vi "Teleop.vi"(10 "Match Info":T1={"Autonomous Elapsed Seconds"=0.0, "TeleOp Elapsed Seconds"=0.0, "Disabled Elapsed Seconds"=0.0, "Visited Autonomous"=FALSE, "Visited TeleOp"=FALSE, "Visited Disabled"=FALSE, "Autonomous Settings"={"Autonomous Style"=enum."Independent", "VI Refnum"=refnum}}, 11 "Call Context":T2) -> ()   [LabVIEW 2014]
doc: "This VI is called for each TeleOp packet received from the DS where the robot is not disabled. It is often used to read from the joysticks and update I/O or to update setpoints for timed control loops. It should complete and return within 20 milliseconds or it may miss DS packets."
uses:
  <vilib>/Rock Robotics/WPI/DriverStation/WPI_DriverStationDerivedRobotMode.ctl
  <vilib>/Rock Robotics/WPI/DriverStation/WPI_DriverStationMatch Info.ctl
  <vilib>/Rock Robotics/WPI/RobotDrive/WPI_RobotDriveGetSetRefNum.vi
  <vilib>/Rock Robotics/WPI/Joystick/WPI_JoystickGetSetRefNum.vi
  <vilib>/Rock Robotics/Network Tables/SD Write Boolean Array.vi
  <vilib>/Rock Robotics/Network Tables/SD Write Numeric Array.vi
  <vilib>/Rock Robotics/Network Tables/SD Write Number.vi
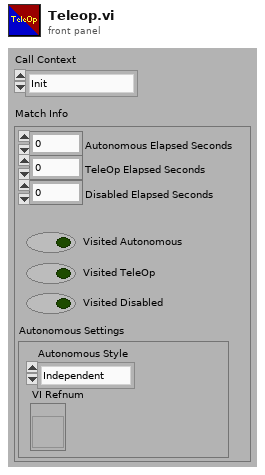
[diagram p1: front panel]
types:
  T1 = typedef "WPI_DriverStationMatch Info.ctl" = cluster{"Autonomous Elapsed Seconds":dbl, "TeleOp Elapsed Seconds":dbl, "Disabled Elapsed Seconds":dbl, "Visited Autonomous":bool, "Visited TeleOp":bool, "Visited Disabled":bool, "Autonomous Settings":cluster{"Autonomous Style":enum16{"Iterative", "Independent"}, "VI Refnum":refnum<vi>}}
  T2 = typedef "WPI_DriverStationDerivedRobotMode.ctl" = enum16{"Init", "Execute", "Stop"}
  T3 = typedef "WPI_MotorControlDeviceRef.ctl" = cluster{"DeviceStatus":errorcluster, "Type":T4, "PWM":cluster{"Controller":T5, "PWM Channel":T6, "DeadBand":T7}, "CAN":cluster{"Device Number":u8, "Control Mode":T8, "Semaphore":T9, "Max Vout":dbl, "TalonSRX Control Mode":T10}, "Invert":bool, "TransformRef":T11, "InvTransformRef":T11}
  T4 = typedef "WPI_MotorControlType.ctl" = enum16{"PWM", "CAN", "CANTalonSRX"}
  T5 = typedef "FPGA_TypedefDigitalModule.ctl" = enum16{"Controller 1"}
  T6 = typedef "FPGA_DIOPWMChannel.ctl" = enum8{"PWM 0", "PWM 1", "PWM 2", "PWM 3", "PWM 4", "PWM 5", "PWM 6", "PWM 7", "PWM 8", "PWM 9", "PWM MXP 0", "PWM MXP 1", "PWM MXP 2", "PWM MXP 3", "PWM MXP 4", "PWM MXP 5", "PWM MXP 6", "PWM MXP 7", "PWM MXP 8", "PWM MXP 9", "Invalid"}
  T7 = typedef "WPI_PWMDeadband.ctl" = cluster{"Name":string, "maxPositivePwm":i32, "minPositivePwm":i32, "centerPwm":i32, "maxNegativePwm":i32, "minNegativePwm":i32, "angularRange":u16}
  T8 = typedef "WPI_CANJaguar_ControlMode.ctl" = enum8{"Percent VBus", "Current", "Speed", "Position", "Voltage"}
  T9 = typedef "Semaphore RefNum" = refnum<k1>
  T10 = typedef "WPI_CANTalonSRX_APIControlMode.ctl" = enum8{"Percent VBus", "Speed", "Position", "Slave", "Unchanged / Invalid"}
  T11 = typedef "WPI_PWMTransform_ConPane.ctl" = refnum<vi>
  T12 = typedef "WPI_JoystickDevRef.ctl" = cluster{"Device":T13}
  T13 = typedef "WPI_JoystickDeviceEnum.ctl" = enum16{"USB 0", "USB 1", "USB 2", "USB 3", "USB 4", "USB 5"}
  T14 = typedef "WPI_RobotDriveDevRef.ctl" = cluster{"DevStatus":errorcluster, "Motors[]":T3[], "Square Inputs":bool, "Max Output":dbl}
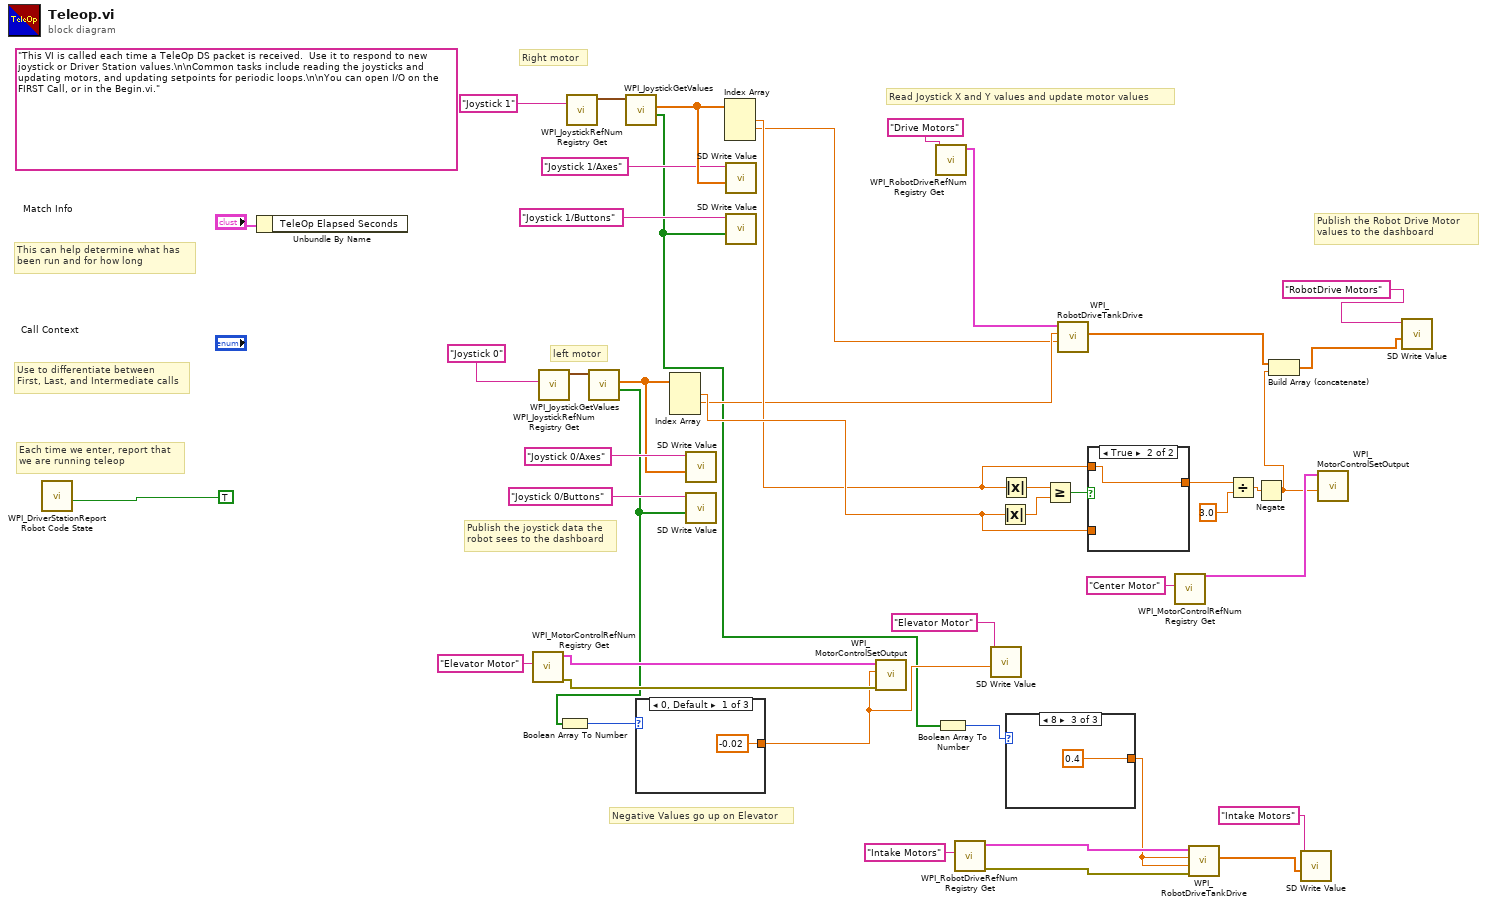
[diagram p0: block diagram]
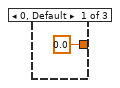
[diagram p2: hidden frame]
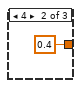
[diagram p3: hidden frame]
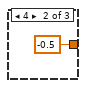
[diagram p4: hidden frame]
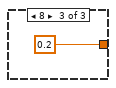
[diagram p5: hidden frame]
diagram:
  (unwired) "This VI is called each time a TeleOp DS packet is received.  Use it to respond to new joystick or Driver Station values.\n\nCommon tasks include reading the joysticks and updating motors, and updating setpoints for periodic loops.\n\nYou can open I/O on the FIRST Call, or in the Begin.vi."
  # "Negative Values go up on Elevator"
  # "left motor"
  # "Right motor"
  # "Publish the Robot Drive Motor\nvalues to the dashboard"
  # "Publish the joystick data the\nrobot sees to the dashboard"
  # "Each time we enter, report that\nwe are running teleop"
  # "Use to differentiate between\nFirst, Last, and Intermediate calls"
  # "This can help determine what has\nbeen run and for how long"
  # "Read Joystick X and Y values and update motor values"
  n1 = call <vilib>:"WPI_DriverStationReport Robot Code State.vi"("TeleOp"=TRUE ("Autonomous")) -> ()  [unwired: 10 in, 1 out]
  n2 = Unbundle By Name("Match Info") -> ()  [unwired: 1 out]
  n3 = call <vilib>:"WPI_MotorControlRefNum Registry Get.vi"("refnum name"="Elevator Motor") -> ("error out"=w19:errorcluster, "MotorControlDevRef"=w20:T3)  [unwired: 9 in]
  n4 = call <vilib>:"WPI_JoystickRefNum Registry Get.vi"("refnum name"="Joystick 0") -> ("JoystickDevRef"=w36:T12)  [unwired: 1 in, 9 out]
  n5 = call <vilib>:"WPI_JoystickRefNum Registry Get.vi"("refnum name"="Joystick 1") -> ("JoystickDevRef"=w31:T12)  [unwired: 9 in, 1 out]
  n6 = call <vilib>:"WPI_JoystickGetValues.vi"("JoystickDevRef"=w36) -> ("Buttons"=w18:bool[], "Axes"=w38:dbl[])  [unwired: 6 in, 3 out]
  n7 = Boolean Array To Number(Boolean array=w18) -> (number=w17:u32)
  n8 = call <vilib>:"WPI_JoystickGetValues.vi"("JoystickDevRef"=w31) -> ("Buttons"=w5:bool[], "Axes"=w35:dbl[])  [unwired: 6 in, 3 out]
  n9 = case shown="0, Default" w17 {
    tunnel: [-0.02 ("Output") -0.5 ("Output") 0.2 ("Output")] -> w15
    frame 0, Default {
    }
    frame 4 {
    }
    frame 8 {
    }
  }
  n10 = Index Array(array=w38) -> (element #1=w24:dbl, element #2=w14:dbl)  [unwired: 3 in, 1 out]
  n11 = call-poly <vilib>:"SD Write Value.vi"("Numeric Array"=w38, "Name"="Joystick 0/Axes") -> ()  [unwired: 8 in, 2 out]
  n12 = call-poly <vilib>:"SD Write Value.vi"("Boolean Array"=w18, "Name"="Joystick 0/Buttons") -> ()  [unwired: 8 in, 2 out]
  n13 = Index Array(array=w35) -> (element #1=w23:dbl, element #2=w13:dbl)  [unwired: 3 in, 1 out]
  n14 = call-poly <vilib>:"SD Write Value.vi"("Numeric Array"=w35, "Name"="Joystick 1/Axes") -> ()  [unwired: 8 in, 2 out]
  n15 = call-poly <vilib>:"SD Write Value.vi"("Boolean Array"=w5, "Name"="Joystick 1/Buttons") -> ()  [unwired: 8 in, 2 out]
  n16 = call <vilib>:"WPI_MotorControlSetOutput.vi"("error in (no error)"=w19, "Output"=w15, "MotorControlDevRef"=w20) -> ()  [unwired: 6 in, 3 out]
  n17 = call <vilib>:"WPI_RobotDriveRefNum Registry Get.vi"("refnum name"="Drive Motors") -> ("RobotDriveDevRef"=w22:T14)  [unwired: 1 in, 9 out]
  n18 = Boolean Array To Number(Boolean array=w5) -> (number=w4:u32)
  n19 = call <vilib>:"WPI_RobotDriveRefNum Registry Get.vi"("refnum name"="Intake Motors") -> ("error out"=w7:errorcluster, "RobotDriveDevRef"=w6:T14)  [unwired: 9 in]
  n20 = call-poly <vilib>:"SD Write Value.vi"("Numeric"=w15, "Name"="Elevator Motor") -> ()  [unwired: 8 in, 2 out]
  n21 = Absolute Value(x=w24) -> (abs(x)=w27:dbl)
  n22 = Absolute Value(x=w23) -> (abs(x)=w28:dbl)
  n23 = case shown="8" w4 {
    tunnel: [0.0 ("Output") 0.4 ("Output") 0.4 ("Output")] -> w3
    frame 0, Default {
    }
    frame 4 {
    }
    frame 8 {
    }
  }
  n24 = Greater Or Equal?(x=w28, y=w27) -> (x >= y?=w29:bool)
  n25 = call <vilib>:"WPI_RobotDriveTankDrive.vi"("Right axis value"=w13, "Left axis value"=w14, "RobotDriveDevRef"=w22) -> ("Motor Values"=w11:dbl[])  [unwired: 6 in, 2 out]
  n26 = case shown="True" w29 {
    tunnel: [w52 w53] -> w12
    tunnel: w23 -> [_ w53]
    tunnel: w24 -> [w52 _]
    frame False {
    }
    frame True {
    }
  }
  n27 = call <vilib>:"WPI_MotorControlRefNum Registry Get.vi"("refnum name"="Center Motor") -> ("MotorControlDevRef"=w39:T3)  [unwired: 9 in, 1 out]
  n28 = call <vilib>:"WPI_RobotDriveTankDrive.vi"("error in (no error)"=w7, "Right axis value"=w3, "Left axis value"=w3, "RobotDriveDevRef"=w6) -> ("Motor Values"=w1:dbl[])  [unwired: 5 in, 2 out]
  n29 = Divide(x=w12, y=3.0) -> (x/y=w25:dbl)
  n30 = Negate(x=w25) -> (-x=w9:dbl)
  n31 = Build Array (concatenate)(w11, w9) -> (w10:dbl[])
  n32 = call-poly <vilib>:"SD Write Value.vi"("Numeric Array"=w1, "Name"="Intake Motors") -> ()  [unwired: 8 in, 2 out]
  n33 = call <vilib>:"WPI_MotorControlSetOutput.vi"("Output"=w9, "MotorControlDevRef"=w39) -> ()  [unwired: 7 in, 3 out]
  n34 = call-poly <vilib>:"SD Write Value.vi"("Numeric Array"=w10, "Name"="RobotDrive Motors") -> ()  [unwired: 8 in, 2 out]
